vi "DQMH Tester Cleanup hse-appl.vi"(8 "error in":errorcluster, 11 "Stop?":bool) -> (0 "error out":errorcluster)   [LabVIEW 2020, in "hse-dqmh.lvlib"]
doc: "If the hse-application object was instantiated and the hse-logger was initialized when starting the Tester, this VI cleans up both objects.\n\n____\nHAMPEL SOFTWARE ENGINEERING v3.8.0 (2023-12-18 14:41)"
uses:
  hse-dqmh.lvlib
  hse-application/hse-application.lvclass
  <vilib>/Hampel Software Engineering/HSE Logger/hse-logger.lvlib
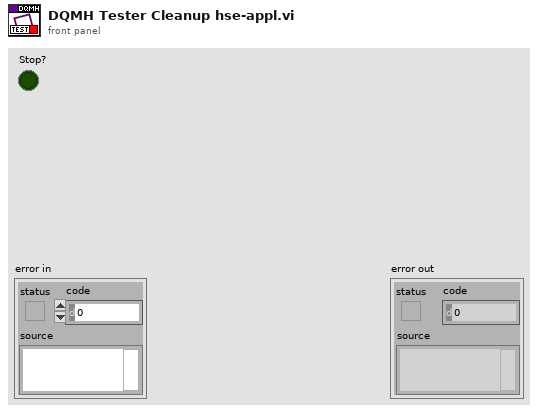
[diagram p1: front panel]
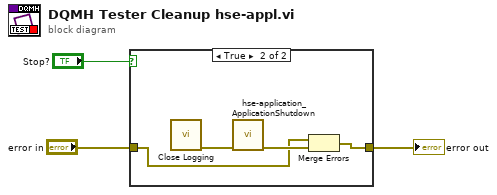
[diagram p0: block diagram]
diagram:
  n1 = case shown="True" "Stop?" {
    tunnel: "error in" -> [w4 w5]
    tunnel: [w4 w6] -> w2
    frame False {
    }
    frame True {
      n2 = call <vilib>:"Close Logging.vi"() -> ("error out"=w8:errorcluster)  [unwired: 11 in]
      n3 = call "hse-application_ApplicationShutdown.vi"("error in"=w8) -> ("error out"=w7:errorcluster)  [unwired: 10 in]
      n4 = Merge Errors(w5, w7) -> (w6:errorcluster)
    }
  }
  "error out" <- w2
